vi "Calculate Job and Machine Orders.vi"(9 "Number of Jobs":i32, 10 "Number of Machines":i32, 11 "Schedule":u16[](array[numeric])) -> (2 "MO4J":u16[][](array[numeric]), 3 "JO4M":u16[][](array[numeric]))   [LabVIEW 2013, in "GA.lvclass"]
uses:
  GA.lvclass
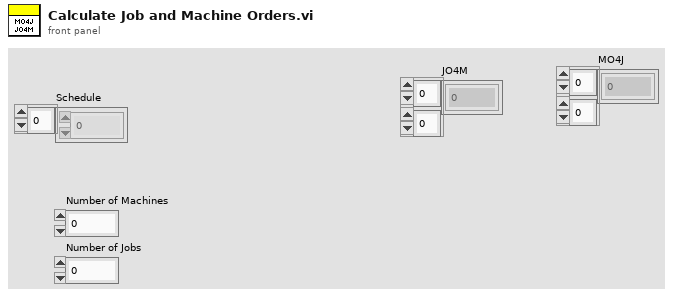
[diagram p1: front panel]
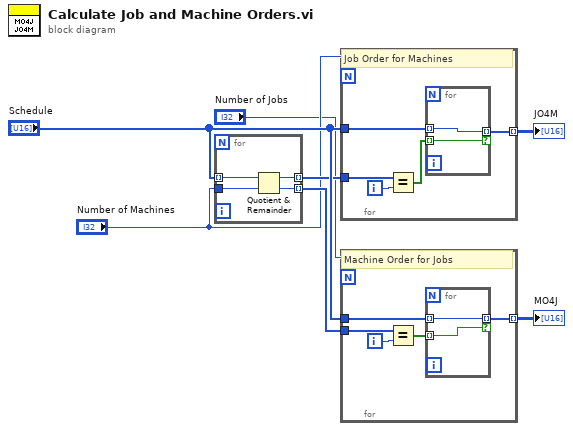
[diagram p0: block diagram]
diagram:
  n1 = for {
    tunnel: "Schedule" -> [w11] mode=indexing
    tunnel: "Number of Machines" -> [w10]
    tunnel: [w9] -> w5 mode=indexing
    tunnel: [w8] -> w6 mode=indexing
    n2 = Quotient & Remainder(x=w11, y=w10) -> (x-y*floor(x/y)=w9:i32, floor(x/y)=w8:i32)
  }
  n3 = for {
    N: "Number of Machines" -> [_]
    tunnel: "Schedule" -> [w14]
    tunnel: w5 -> [w13]
    tunnel: [w12] -> w3 mode=indexing
    i -> [w16]
    # "Job Order for Machines"
    n4 = Equal?(x=w13, y=w16) -> (x = y?=w15:bool[])
    n5 = for {
      tunnel: w15 -> [w18] mode=indexing
      tunnel: [w17] -> w12 mode=indexing if=w18
      tunnel: w14 -> [w17] mode=indexing
    }
  }
  "JO4M" <- w3
  n6 = for {
    N: "Number of Jobs" -> [_]
    tunnel: "Schedule" -> [w21]
    tunnel: [w20] -> w4 mode=indexing
    tunnel: w6 -> [w19]
    i -> [w23]
    # "Machine Order for Jobs"
    n7 = Equal?(x=w19, y=w23) -> (x = y?=w22:bool[])
    n8 = for {
      tunnel: w22 -> [w24] mode=indexing
      tunnel: w21 -> [w25] mode=indexing
      tunnel: [w25] -> w20 mode=indexing if=w24
    }
  }
  "MO4J" <- w4
